vi "FilterEngine.vi"() -> ()   [LabVIEW 2018]
uses:
  classes/Tushars Events Toolkit/Software/Modules/EventClient_ObjectReference.ctl
  Strict Type Controls/Settings Operation.ctl
  classes/Variable Manager/VariableManager_Bool.vi
  <vilib>/Instr/_visa.llb/VISA Configure Serial Port (Instr).vi
  ctrlFilterCommands.ctl
  ctrlMoveDirection.ctl
panel:
  out "isConnected?":bool
  in  "stop":bool
  in  "home":bool
  in  "speed(steps/Sec)":u32=100 min=100 max=10000 step=1
  in  "setSpeed":bool
  in  "Direction":T1 items=["Cloclwise"=175, "Anti-Cloclwise"=125]
  in  "relAngleMove":sgl
  in  "move":bool
  out "Quit":bool
  out "error out":errorcluster
  in  "error in (no error)":errorcluster
  out "remAngle":sgl
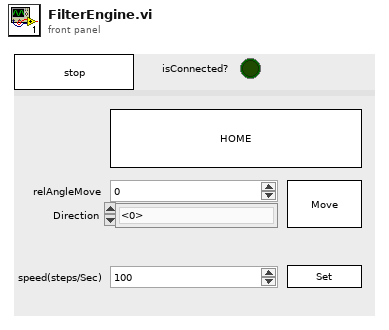
[diagram p1: front panel]
types:
  T1 = typedef "ctrlMoveDirection.ctl" = u8
  T2 = typedef "ctrlFilterCommands.ctl" = u8
  T3 = cluster{"filterPort":refnum<visa-resource-name>, "data":u8[], "bytesForWait":u8[], "filterCmd":T2, "ackBytes":u8[], "currAngle":i32}
  T4 = typedef "EventClient_ObjectReference.ctl" = refnum<k1>
  T5 = typedef "Settings Operation.ctl" = enum8{"Get Value", "Set Value", "Read File", "Write File", "Write Stored Value"}
  T6 = cluster{"Port":refnum<visa-resource-name>, "baud rate":u32, "data bits":u16, "stop bits":u16, "parity":enum16{"None", "Odd", "Even", "Mark", "Space"}, "flow control":u16, "Timeout":u32}
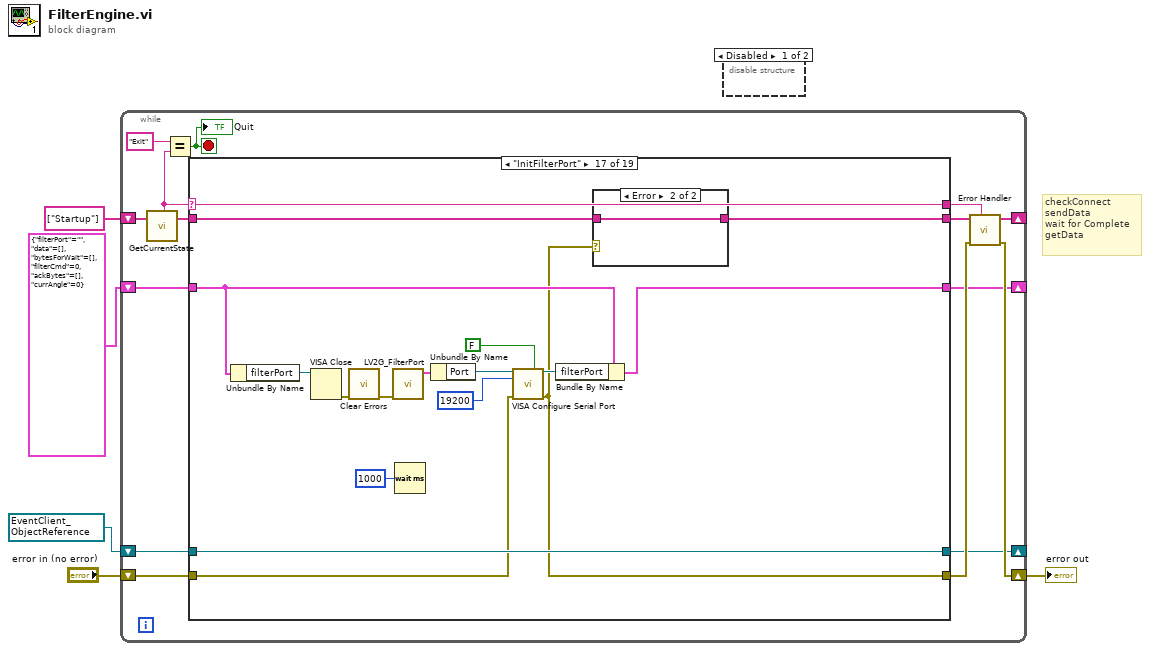
[diagram p0: block diagram]
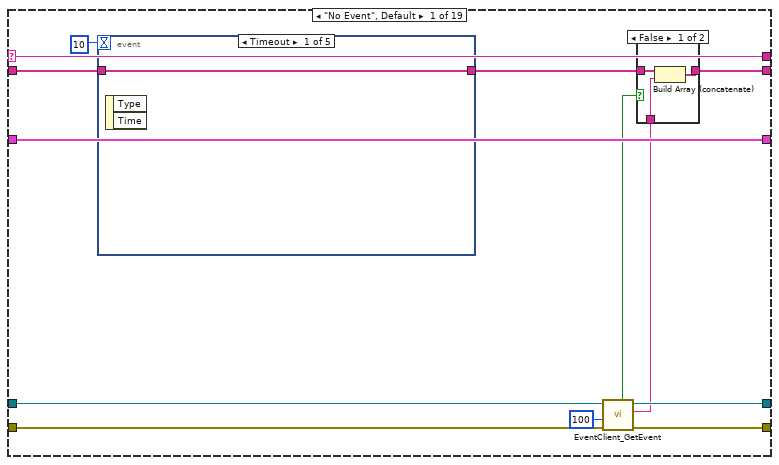
[diagram p3: hidden frame]
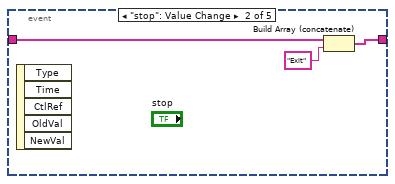
[diagram p5: hidden frame]
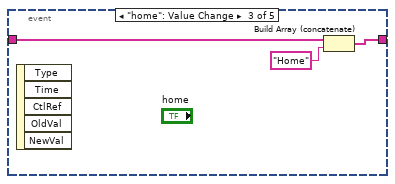
[diagram p6: hidden frame]
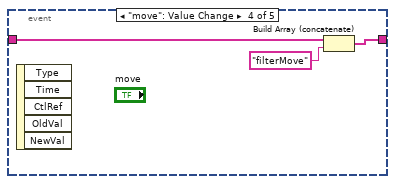
[diagram p7: hidden frame]
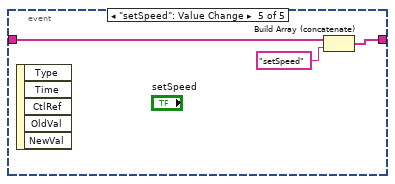
[diagram p8: hidden frame]
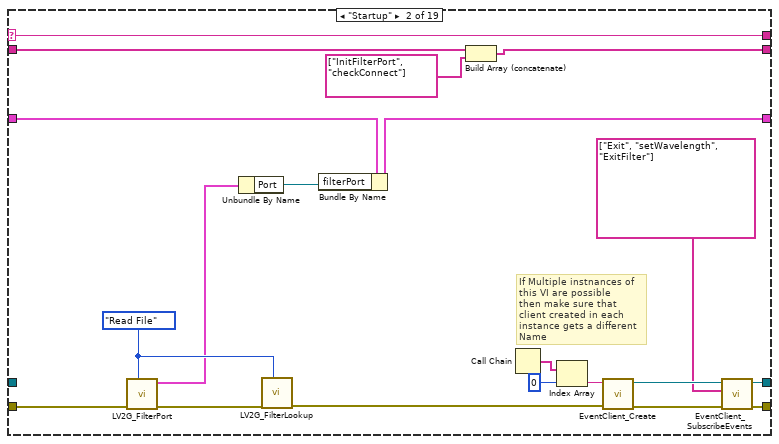
[diagram p9: hidden frame]
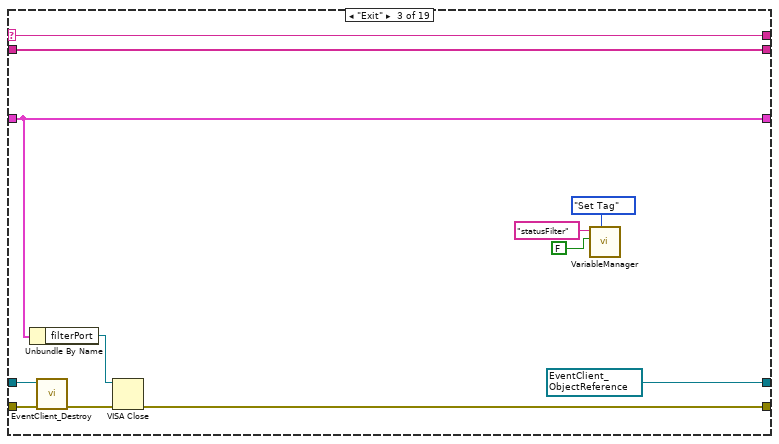
[diagram p10: hidden frame]
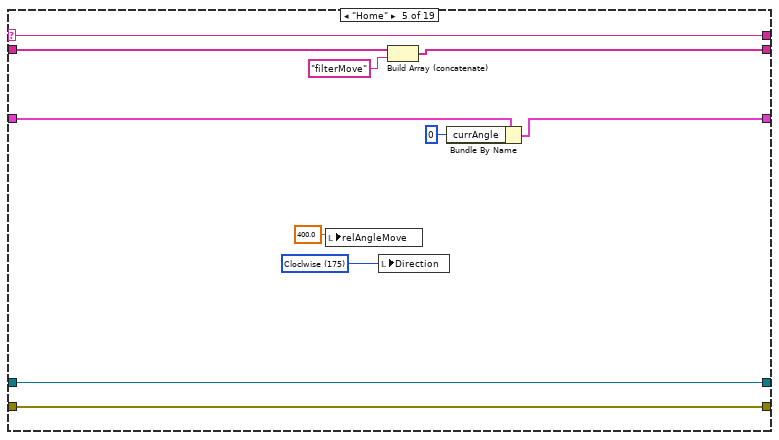
[diagram p12: hidden frame]
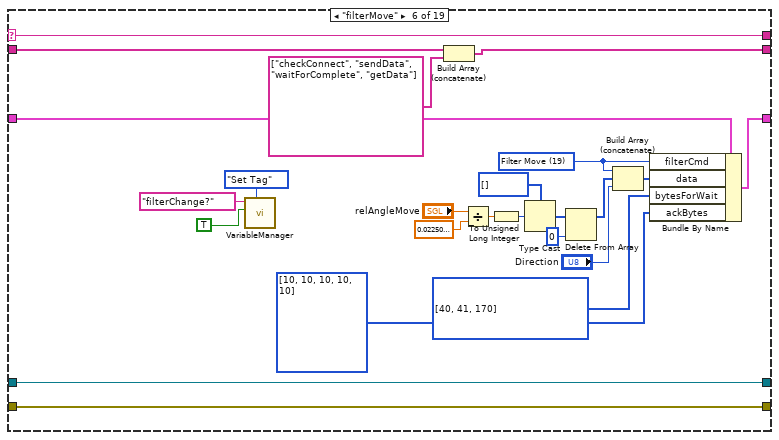
[diagram p13: hidden frame]
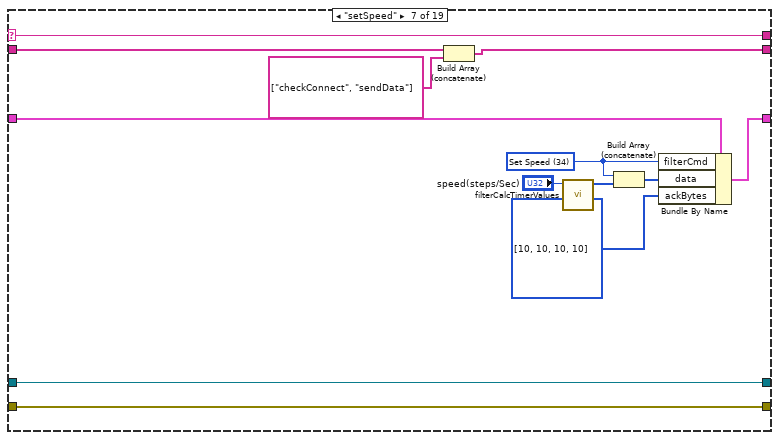
[diagram p14: hidden frame]
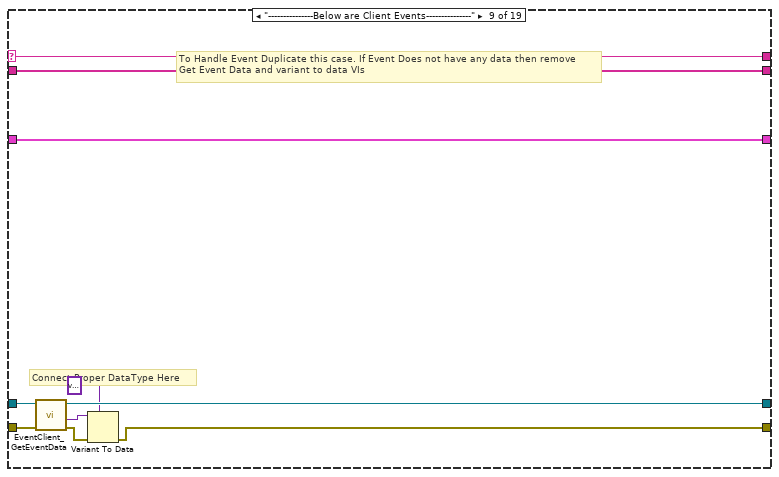
[diagram p16: hidden frame]
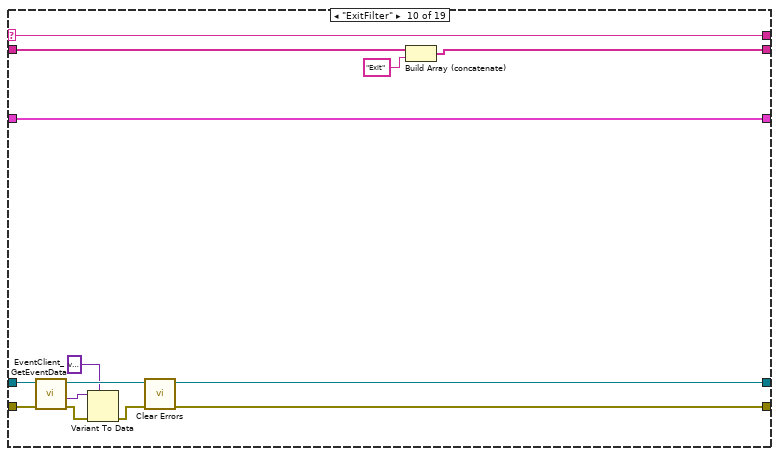
[diagram p17: hidden frame]
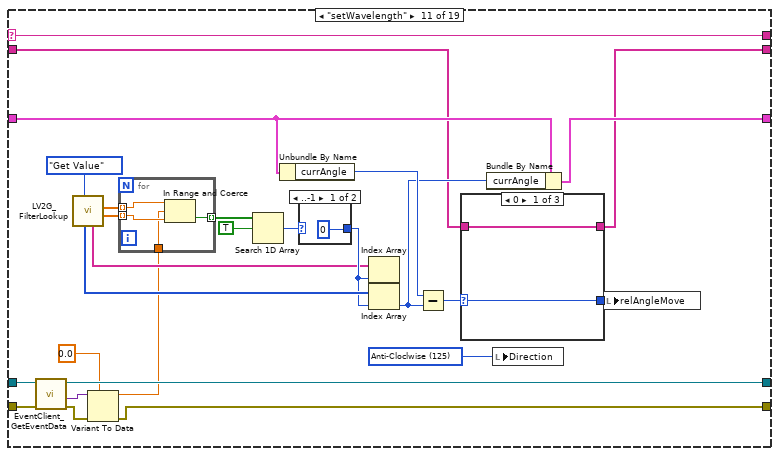
[diagram p18: hidden frame]
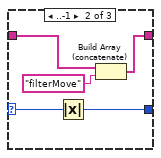
[diagram p19: hidden frame]
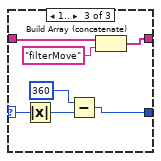
[diagram p20: hidden frame]
diagram:
  w2 = T4 refnum items=["EventClient"] ("reference")
  # "checkConnect\nsendData\nwait for Complete\ngetData"
  n1 = while {
    shift-right: [w16] -> _
    shift-left: string[] ["Startup"] ("State Array Out") -> [w20]
    shift-right: [w12] -> w3
    shift-left: "error in (no error)" -> [w13]
    shift-right: [w9] -> _
    shift-left: w2 -> [w8]
    shift-right: [w7] -> _
    shift-left: T3 {"filterPort"="", "data"=[], "bytesForWait"=[], "filterCmd"=0, "ackBytes"=[], "currAngle"=0} -> [w6]
    stop <- w17 stop-if-true
    n2 = call "GetCurrentState.vi"("State Array In"=w20) -> ("Current State"=w10:string, "State Array Out"=w19:string[])  [unwired: 17 in]
    n3 = Equal?(x="Exit", y=w10) -> (x = y?=w17:bool)
    "Quit" <- w17
    n4 = case shown="\"InitFilterPort\"" w10 {
      selector: w10 -> [w27 w70 w82 w86 w97 w121 w134 w139 w149 w162 w190 w214 w236 w250 w267 w310 w338 w347 w363]
      tunnel: w19 -> [w24 w69 w81 w87 w98 w122 w135 w140 w150 w163 w166 w215 w219 w242 w269 w303 w324 w346 w350]
      tunnel: [w28 w68 w81 w87 w91 w116 w130 w140 w150 w153 w165 w215 w219 w241 w268 w303 w323 w346 w350] -> w15
      tunnel: [w31 w62 w73 w85 w96 w120 w123 w138 w145 w151 w186 w213 w226 w243 w279 w287 w322 w345 errorcluster {"status"=FALSE, "code"=0, "source"=""} ("error in (no error)")] -> w11
      tunnel: [w27 w70 w82 w86 w97 w121 w134 w139 w149 w162 w190 w214 w236 w250 w267 w310 w338 w347 w363] -> w14
      tunnel: w13 -> [w32 w55 w79 w85 w96 w120 w123 w138 w147 w160 w188 w213 w227 w244 w275 w304 w334 w345 w351]
      tunnel: [w30 w60 w78 w84 w95 w119 w133 w137 w143 w156 w184 w212 w235 w249 w281 w309 w337 w344 w349] -> w9
      tunnel: w8 -> [w33 _ w80 w84 w95 w119 w133 w137 w148 w161 w189 w212 w235 w249 w281 w309 w337 w344 w349]
      tunnel: [w26 w56 w72 w83 w89 w118 w132 w136 w141 w154 w169 w211 w233 w247 w270 w307 w335 w343 w348] -> w7
      tunnel: w6 -> [w26 w58 w72 w83 w94 w117 w131 w136 w141 w154 w170 w211 w234 w248 w271 w308 w336 w343 w348]
      frame "No Event", Default {
        n5 = event shown="[0] Timeout" {
          selector: _ -> [_ _ _ _ _]
          dyn-events: _ -> [_ _ _ _ _]
          timeout: 10 -> [_ _ _ _ _]
          tunnel: w24 -> [w38 w41 w44 w47 w50]
          tunnel: [w38 w40 w43 w46 w49] -> w23
          event Timeout {
            n6 = event-data() -> ()  [unwired: 1 in, 2 out]
          }
          event "stop": Value Change {
            n7 = event-data() -> ()  [unwired: 1 in, 5 out]
            n8 = Build Array (concatenate)(w41, "Exit" ("x")) -> (w40:string[])
          }
          event "home": Value Change {
            n9 = event-data() -> ()  [unwired: 1 in, 5 out]
            n10 = Build Array (concatenate)(w44, "Home" ("x")) -> (w43:string[])
          }
          event "move": Value Change {
            n11 = event-data() -> ()  [unwired: 1 in, 5 out]
            n12 = Build Array (concatenate)(w47, "filterMove" ("x")) -> (w46:string[])
          }
          event "setSpeed": Value Change {
            n13 = event-data() -> ()  [unwired: 1 in, 5 out]
            n14 = Build Array (concatenate)(w50, "setSpeed" ("x")) -> (w49:string[])
          }
        }
        n15 = call "EventClient_GetEvent.vi"("error in (no error)"=w32, "timeout in ms (-1)"=100, "reference"=w33) -> ("error out"=w31:errorcluster, "Name"=w21:string, "reference out"=w30:T4, "timed out?"=w22:bool)  [unwired: 4 in, 1 out]
        n16 = case shown="False" w22 {
          tunnel: [w36 w37] -> w28
          tunnel: w23 -> [w35 w37]
          tunnel: w21 -> [w34 _]
          frame False {
            n17 = Build Array (concatenate)(w35, w34) -> (w36:string[])
          }
          frame True {
          }
        }
      }
      frame "Startup" {
        w57 = Settings_Operation."Read File" ("Operation")
        # "If Multiple instnances of this VI are possible \nthen make sure that client created in each instance gets a different Name"
        n18 = call "LV2G_FilterPort.vi"("Operation"=w57, "error in (no error)"=w55) -> ("error out"=w54:errorcluster, "Modbus485 Out"=w52:T6)  [unwired: 8 in]
        n19 = Unbundle By Name(w52) -> ("Port"=w51:refnum<visa-resource-name>)
        n20 = call "LV2G_FilterLookup.vi"("Operation"=w57, "error in (no error)"=w54) -> ("error out"=w53:errorcluster)  [unwired: 4 in, 5 out]
        n21 = Bundle By Name(cluster=w58, "filterPort"=w51) -> (w56:T3)
        n22 = Build Array (concatenate)(w69, string[] ["InitFilterPort", "checkConnect"] ("State Array Out")) -> (w68:string[])
        n23 = Call Chain() -> (call chain=w66:string[])
        n24 = Index Array(array=w66, index=0) -> (element=w64:string)
        n25 = call "EventClient_Create.vi"("error in (no error)"=w53, "Instance Name"=w64) -> ("error out"=w63:errorcluster, "reference"=w61:T4)  [unwired: 8 in]
        n26 = call "EventClient_SubscribeEvents.vi"("error in (no error)"=w63, "Events"=string[] ["Exit", "setWavelength", "ExitFilter"], "reference"=w61) -> ("error out"=w62:errorcluster, "reference out"=w60:T4)  [unwired: 7 in]
      }
      frame "Exit" {
        w78 = T4 refnum items=["EventClient"] ("reference out")
        n27 = Unbundle By Name(w72) -> ("filterPort"=w75:refnum<visa-resource-name>)
        n28 = call "EventClient_Destroy.vi"("error in (no error)"=w79, "reference"=w80) -> ("error out"=w74:errorcluster)  [unwired: 9 in]
        n29 = VISA Close(VISA resource name=w75, error in (no error)=w74) -> (error out=w73:errorcluster)
        n30 = call-poly "VariableManager.vi"("Operation"=enum16{"Get Tag", "Set Tag"}."Set Tag", "Value"=FALSE, "Tag"="statusFilter") -> ()  [unwired: 5 in, 4 out]
      }
      frame "---------------Below are UI Events---------------" {
        # "This State will never Execute\nIt is added just for improving code readability please do not remove this case"
      }
      frame "Home" {
        w92 = T1 175 items=["Cloclwise"=175, "Anti-Cloclwise"=125] ("filterMoveDirection")
        n31 = local write "relAngleMove"(sgl 400.0 ("deg")) -> ()
        n32 = local write "Direction"(w92) -> ()
        n33 = Build Array (concatenate)(w98, "filterMove") -> (w91:string[])
        n34 = Bundle By Name(cluster=w94, "currAngle"=0) -> (w89:T3)
      }
      frame "filterMove" {
        w102 = T2[] [10, 10, 10, 10, 10] items=["ACK"=10, "Filter Move"=19, "Set Speed"=34, "X Limit 1"=40, "X limit 2"=41, "Connect"=100, "STOP"=104, "STOP ACK"=105, "Get Readings"=163, "Get Readings ACK"=164, "Move Complete"=170, "TriggerIN"=187, "Trigger ACK"=191, "TriggerOUT"=192, "Connect ACK"=200]
        w106 = T2[] [40, 41, 170] items=["ACK"=10, "Filter Move"=19, "Set Speed"=34, "X Limit 1"=40, "X limit 2"=41, "Connect"=100, "STOP"=104, "STOP ACK"=105, "Get Readings"=163, "Get Readings ACK"=164, "Move Complete"=170, "TriggerIN"=187, "Trigger ACK"=191, "TriggerOUT"=192, "Connect ACK"=200]
        w104 = T2 19 items=["ACK"=10, "Filter Move"=19, "Set Speed"=34, "X Limit 1"=40, "X limit 2"=41, "Connect"=100, "STOP"=104, "STOP ACK"=105, "Get Readings"=163, "Get Readings ACK"=164, "Move Complete"=170, "TriggerIN"=187, "Trigger ACK"=191, "TriggerOUT"=192, "Connect ACK"=200] ("filterCmd")
        n35 = call-poly "VariableManager.vi"("Operation"=enum16{"Get Tag", "Set Tag"}."Set Tag", "Value"=TRUE, "Tag"="filterChange?") -> ()  [unwired: 5 in, 4 out]
        n36 = Build Array (concatenate)(w122, string[] ["checkConnect", "sendData", "waitForComplete", "getData"]) -> (w116:string[])
        n37 = Divide(x="relAngleMove", y=sgl 0.0225) -> (x/y=w112:sgl)
        n38 = To Unsigned Long Integer(number=w112) -> (unsigned 32bit integer=w111:u32)
        n39 = Type Cast(type=u8[] [], x=w111) -> (*(type *) &x=w109:u8[])
        n40 = Delete From Array(array=w109, index=0) -> (array with subset deleted=w107:u8[])  [unwired: 1 in, 1 out]
        n41 = Build Array (concatenate)(w104, w107, "Direction") -> (w105:T1[])
        n42 = Bundle By Name(cluster=w117, "filterCmd"=w104, "data"=w105, "bytesForWait"=w106, "ackBytes"=w102) -> (w118:T3)
      }
      frame "setSpeed" {
        w126 = T2[] [10, 10, 10, 10] items=["ACK"=10, "Filter Move"=19, "Set Speed"=34, "X Limit 1"=40, "X limit 2"=41, "Connect"=100, "STOP"=104, "STOP ACK"=105, "Get Readings"=163, "Get Readings ACK"=164, "Move Complete"=170, "TriggerIN"=187, "Trigger ACK"=191, "TriggerOUT"=192, "Connect ACK"=200]
        w127 = T2 34 items=["ACK"=10, "Filter Move"=19, "Set Speed"=34, "X Limit 1"=40, "X limit 2"=41, "Connect"=100, "STOP"=104, "STOP ACK"=105, "Get Readings"=163, "Get Readings ACK"=164, "Move Complete"=170, "TriggerIN"=187, "Trigger ACK"=191, "TriggerOUT"=192, "Connect ACK"=200] ("filterCmd")
        n43 = Build Array (concatenate)(w135, string[] ["checkConnect", "sendData"]) -> (w130:string[])
        n44 = call "filterCalcTimerValues.vi"("speed(steps/Sec)"="speed(steps/Sec)") -> ("data"=w124:u8[])  [unwired: 8 in, 2 out]
        n45 = Build Array (concatenate)(w127, w124) -> (w128:T2[])
        n46 = Bundle By Name(cluster=w131, "filterCmd"=w127, "data"=w128, "ackBytes"=w126) -> (w132:T3)
      }
      frame "---------------Below are Menu Events---------------" {
        # "This State will never Execute\nIt is added just for improving code readability please do not remove this case"
      }
      frame "---------------Below are Client Events---------------" {
        # "To Handle Event Duplicate this case. If Event Does not have any data then remove\nGet Event Data and variant to data VIs"
        # "Connect Proper DataType Here"
        n47 = call "EventClient_GetEventData.vi"("error in (no error)"=w147, "reference"=w148) -> ("error out"=w146:errorcluster, "Data"=w144:variant, "reference out"=w143:T4)  [unwired: 7 in]
        n48 = Variant To Data(error in=w146, type=variant, Variant=w144) -> (error out=w145:errorcluster)  [unwired: 1 out]
      }
      frame "ExitFilter" {
        n49 = call "EventClient_GetEventData.vi"("error in (no error)"=w160, "reference"=w161) -> ("error out"=w159:errorcluster, "Data"=w157:variant, "reference out"=w156:T4)  [unwired: 7 in]
        n50 = Variant To Data(error in=w159, type=variant, Variant=w157) -> (error out=w158:errorcluster)  [unwired: 1 out]
        n51 = call <vilib>:"Clear Errors.vi"("error in (no error)"=w158) -> ("error out"=w151:errorcluster)  [unwired: 5 in, 1 out]
        n52 = Build Array (concatenate)(w163, "Exit" ("x")) -> (w153:string[])
      }
      frame "setWavelength" {
        w171 = T1 125 items=["Cloclwise"=175, "Anti-Cloclwise"=125] ("filterMoveDirection")
        n53 = call "EventClient_GetEventData.vi"("error in (no error)"=w188, "reference"=w189) -> ("error out"=w187:errorcluster, "Data"=w185:variant, "reference out"=w184:T4)  [unwired: 7 in]
        n54 = call "LV2G_FilterLookup.vi"("Operation"=Settings_Operation."Get Value") -> ("minRange"=w180:dbl[], "maxRange"=w181:dbl[], "filters"=w174:string[], "angles"=w176:i32[])  [unwired: 5 in, 2 out]
        n55 = Variant To Data(error in=w187, type=0.0 ("wavelength"), Variant=w185) -> (data=w173:dbl, error out=w186:errorcluster)
        n56 = for {
          tunnel: w181 -> [w210] mode=indexing
          tunnel: w180 -> [w209] mode=indexing
          tunnel: [w208] -> w179 mode=indexing
          tunnel: w173 -> [w207]
          n57 = In Range and Coerce(upper limit=w210, x=w207, lower limit=w209) -> (In Range?=w208:bool)  [unwired: 1 out]
        }
        n58 = Search 1D Array(1D array=w179, element=TRUE) -> (index of element=w177:i32)  [unwired: 1 in]
        n59 = Unbundle By Name(w170) -> ("currAngle"=w172:i32)
        n60 = case shown="..-1" w177 {
          selector: w177 -> [_ w206]
          tunnel: [0 ("index of element") w206] -> w175
          frame ..-1 {
          }
          frame 0.. {
          }
        }
        n61 = Index Array(array=w174, index=w175) -> ()  [unwired: 1 out]
        n62 = Index Array(array=w176, index=w175) -> (element=w168:i32)
        n63 = Subtract(x=w172, y=w168) -> (x-y=w167:i32)
        n64 = case shown="0" w167 {
          selector: w167 -> [w191 w196 w204]
          tunnel: w166 -> [w192 w197 w199]
          tunnel: [w192 w194 w198] -> w165
          tunnel: [w191 w195 w201] -> w164
          frame 0 {
          }
          frame ..-1 {
            n65 = Absolute Value(x=w196) -> (abs(x)=w195:i32)
            n66 = Build Array (concatenate)(w197, "filterMove" ("x")) -> (w194:string[])
          }
          frame 1.. {
            n67 = Absolute Value(x=w204) -> (abs(x)=w202:i32)
            n68 = Subtract(x=360, y=w202) -> (x-y=w201:i32)
            n69 = Build Array (concatenate)(w199, "filterMove" ("x")) -> (w198:string[])
          }
        }
        n70 = Bundle By Name(cluster=w170, "currAngle"=w168) -> (w169:T3)
        n71 = local write "Direction"(w171) -> ()
        n72 = local write "relAngleMove"(w164) -> ()
      }
      frame "---------------Below are Subroutine states---------------" {
      }
      frame "checkConnect" {
        w220 = T2 200 items=["ACK"=10, "Filter Move"=19, "Set Speed"=34, "X Limit 1"=40, "X limit 2"=41, "Connect"=100, "STOP"=104, "STOP ACK"=105, "Get Readings"=163, "Get Readings ACK"=164, "Move Complete"=170, "TriggerIN"=187, "Trigger ACK"=191, "TriggerOUT"=192, "Connect ACK"=200] ("filterCmd")
        w224 = T2 100 items=["ACK"=10, "Filter Move"=19, "Set Speed"=34, "X Limit 1"=40, "X limit 2"=41, "Connect"=100, "STOP"=104, "STOP ACK"=105, "Get Readings"=163, "Get Readings ACK"=164, "Move Complete"=170, "TriggerIN"=187, "Trigger ACK"=191, "TriggerOUT"=192, "Connect ACK"=200] ("filterCmd")
        n73 = Unbundle By Name(w234) -> ("filterPort"=w229:refnum<visa-resource-name>)
        n74 = Type Cast(x=w224) -> (*(type *) &x=w225:string)  [unwired: 1 in]
        n75 = VISA Write(VISA resource name=w229, write buffer=w225, error in (no error)=w227) -> (VISA resource name out=w232:refnum<visa-resource-name>, error out=w228:errorcluster)  [unwired: 1 out]
        n76 = call "filterReadTimeout.vi"("error in (no error)"=w228, "timeoutMs"=u32 100, "filterPort"=w232) -> ("error out"=w226:errorcluster, "rxData"=w223:string, "filterPortOut"=w230:refnum<visa-resource-name>)  [unwired: 6 in]
        n77 = Type Cast(type=u8 0, x=w223) -> (*(type *) &x=w221:u8)
        n78 = Bundle By Name(cluster=w234, "filterPort"=w230) -> (w233:T3)
        n79 = Equal?(x=w221, y=w220) -> (x = y?=w216:bool)
        "isConnected?" <- w216
        n80 = call-poly "VariableManager.vi"("Operation"=enum16{"Get Tag", "Set Tag"}."Set Tag", "Value"=w216, "Tag"="statusFilter") -> ()  [unwired: 5 in, 4 out]
      }
      frame "sendData" {
        n81 = Unbundle By Name(w248) -> ("filterPort"=w245:refnum<visa-resource-name>, "data"=w238:u8[], "ackBytes"=w237:u8[])
        n82 = for {
          tunnel: w244 -> [w261]
          tunnel: [w260] -> w243
          tunnel: [w259] -> w240 mode=indexing
          tunnel: w238 -> [w252] mode=indexing
          tunnel: w237 -> [w251] mode=indexing
          shift-right: [w263] -> w246
          shift-left: w245 -> [w262]
          n83 = Type Cast(x=w252) -> (*(type *) &x=w255:string)  [unwired: 1 in]
          n84 = Type Cast(x=w251) -> (*(type *) &x=w253:string)  [unwired: 1 in]
          n85 = VISA Write(VISA resource name=w262, write buffer=w255, error in (no error)=w261) -> (VISA resource name out=w258:refnum<visa-resource-name>, error out=w256:errorcluster)  [unwired: 1 out]
          n86 = call "filterReadTimeout.vi"("error in (no error)"=w256, "matchChar"=w253, "timeoutMs"=u32 100, "filterPort"=w258) -> ("error out"=w260:errorcluster, "rxData"=w254:string, "filterPortOut"=w263:refnum<visa-resource-name>)  [unwired: 5 in]
          n87 = Equal?(x=w254, y=w253) -> (x = y?=w259:bool)
        }
        n88 = And Array Elements(Boolean array=w240) -> (logical AND=w239:bool)
        n89 = case shown="False" w239 {
          tunnel: w242 -> [_ w265]
          tunnel: [string[] [] ("State Array Out") w265] -> w241
          frame False {
          }
          frame True {
          }
        }
        n90 = Bundle By Name(cluster=w248, "filterPort"=w246) -> (w247:T3)
      }
      frame "waitForComplete" {
        n91 = Unbundle By Name(w271) -> ("filterPort"=w276:refnum<visa-resource-name>, "bytesForWait"=w274:u8[])
        n92 = call "filterReadTimeout.vi"("error in (no error)"=w275, "timeoutMs"=u32 100, "filterPort"=w276) -> ("error out"=w279:errorcluster, "rxData"=w278:string, "filterPortOut"=w272:refnum<visa-resource-name>)  [unwired: 6 in]
        n93 = Type Cast(type=u8 0, x=w278) -> (*(type *) &x=w273:u8)
        n94 = Search 1D Array(1D array=w274, element=w273) -> (index of element=w266:i32)  [unwired: 1 in]
        n95 = case shown="0.." w266 {
          tunnel: w269 -> [w282 w285]
          tunnel: [w282 w284] -> w268
          tunnel: w267 -> [_ w283]
          frame 0.. {
          }
          frame ..-1 {
            n96 = Build Array (concatenate)(w283, w285) -> (w284:string[])
          }
        }
        n97 = Bundle By Name(cluster=w271, "filterPort"=w272) -> (w270:T3)
      }
      frame "getData" {
        w301 = T2 164 items=["ACK"=10, "Filter Move"=19, "Set Speed"=34, "X Limit 1"=40, "X limit 2"=41, "Connect"=100, "STOP"=104, "STOP ACK"=105, "Get Readings"=163, "Get Readings ACK"=164, "Move Complete"=170, "TriggerIN"=187, "Trigger ACK"=191, "TriggerOUT"=192, "Connect ACK"=200] ("filterCmd")
        w302 = T2[] [163, 10, 10, 10] items=["ACK"=10, "Filter Move"=19, "Set Speed"=34, "X Limit 1"=40, "X limit 2"=41, "Connect"=100, "STOP"=104, "STOP ACK"=105, "Get Readings"=163, "Get Readings ACK"=164, "Move Complete"=170, "TriggerIN"=187, "Trigger ACK"=191, "TriggerOUT"=192, "Connect ACK"=200]
        n98 = Unbundle By Name(w308) -> ("filterPort"=w305:refnum<visa-resource-name>)
        n99 = Type Cast(x=w301) -> (*(type *) &x=w300:string)  [unwired: 1 in]
        n100 = for {
          tunnel: w304 -> [w316]
          tunnel: [w315] -> w287
          shift-right: [w319] -> w306
          shift-left: w305 -> [w318]
          tunnel: w302 -> [w313] mode=indexing
          tunnel: [w312] -> w299 mode=indexing
          tunnel: w300 -> [w311]
          n101 = Type Cast(x=w313) -> (*(type *) &x=w314:string)  [unwired: 1 in]
          n102 = VISA Write(VISA resource name=w318, write buffer=w314, error in (no error)=w316) -> (VISA resource name out=w321:refnum<visa-resource-name>, error out=w317:errorcluster)  [unwired: 1 out]
          n103 = call "filterReadTimeout.vi"("error in (no error)"=w317, "matchChar"=w311, "timeoutMs"=u32 100, "filterPort"=w321) -> ("error out"=w315:errorcluster, "rxData"=w312:string, "filterPortOut"=w319:refnum<visa-resource-name>)  [unwired: 5 in]
        }
        n104 = Delete From Array(array=w299, index=0) -> (array with subset deleted=w297:string[])  [unwired: 1 in, 1 out]
        n105 = call <vilib>:"Clear Errors.vi"("error in (no error)"=w287) -> ("error out"=w286:errorcluster)  [unwired: 5 in, 1 out]
        n106 = Hexadecimal String To Number(string=w297, default (0uL)=u8 0 ("default (0 U32)")) -> (number=w295:u8[])  [unwired: 1 in, 1 out]
        n107 = Type Cast(type=u32 0, x=w295) -> (*(type *) &x=w293:u32)
        n108 = call-poly "VariableManager.vi"("Operation"=enum16{"Get Tag", "Set Tag"}."Set Tag", "error in (no error)"=w286, "Value"=FALSE, "Tag"="filterChange?") -> ()  [unwired: 4 in, 4 out]
        n109 = Multiply(x=w293, y=sgl 0.0225) -> (x*y=→"remAngle":sgl)
        n110 = Bundle By Name(cluster=w308, "filterPort"=w306) -> (w307:T3)
      }
      frame "InitFilterPort" {
        n111 = Unbundle By Name(w336) -> ("filterPort"=w332:refnum<visa-resource-name>)
        n112 = VISA Close(VISA resource name=w332) -> (error out=w331:errorcluster)  [unwired: 1 in]
        n113 = call <vilib>:"Clear Errors.vi"("error in (no error)"=w331) -> ("error out"=w330:errorcluster)  [unwired: 5 in, 1 out]
        n114 = call "LV2G_FilterPort.vi"("error in (no error)"=w330) -> ("Modbus485 Out"=w329:T6)  [unwired: 9 in, 1 out]
        n115 = Wait (ms)(milliseconds to wait=u32 1000) -> ()  [unwired: 1 out]
        n116 = Unbundle By Name(w329) -> ("Port"=w328:refnum<visa-resource-name>)
        n117 = call-poly "VISA Configure Serial Port"("VISA resource name"=w328, "Enable Termination\nChar (T)"=FALSE ("Enable Termination\nChar (T)"), "baud rate (9600)"=u32 19200, "error in (no error)"=w334) -> ("VISA resource name out"=w325:refnum<visa-resource-name>, "error out"=w322:errorcluster)  [unwired: 10 in]
        n118 = Bundle By Name(cluster=w336, "filterPort"=w325) -> (w335:T3)
        n119 = case shown="Error" w322 {
          tunnel: w324 -> [w341 w342]
          tunnel: [w340 w342] -> w323
          frame No Error {
            n120 = Build Array (concatenate)(w341, "Home") -> (w340:string[])
          }
          frame Error {
          }
        }
      }
      frame "---------------Below are Error Handling VIs---------------" {
      }
      frame "Error" {
        n121 = Call Chain() -> (call chain=w358:string[])
        n122 = for {
          tunnel: w358 -> [w366] mode=indexing
          shift-right: [w364] -> w355
          shift-left: "" -> [w367]
          n123 = Concatenate Strings(w367, w366, " -> ") -> (w364:string)
        }
        n124 = Unbundle By Name(w351) -> ("code"=w353:i32, "source"=w352:string)
        n125 = Match Pattern(string=w352, regular expression=":") -> (before substring=w356:string, after substring=w360:string)  [unwired: 1 in, 2 out]
        n126 = Format Into String(format string="Error Occured In\"%s\" state of \"%s\" VI\nError Code: %d\nError Description: \"%s\"", w356, w355, w353, w360) -> (resulting string=w359:string)  [unwired: 2 in, 1 out]
        n127 = One Button Dialog(message=w359) -> ()  [unwired: 1 in, 1 out]
      }
    }
    n128 = call "Error Handler.vi"("Current State"=w14, "error in (no error)"=w11, "Msg Queue In"=w15) -> ("error out"=w12:errorcluster, "Msg Queue Out"=w16:string[])  [unwired: 7 in]
  }
  "error out" <- w3
  n129 = disable-structure shown="Disabled" {
    frame Disabled {
    }
    frame Enabled {
    }
  }
